vi "rpc_tsmaster_cmd_read_system_var.vi"(8 "error in (no error)":errorcluster caption="Incorrect input (no errors)", 9 "AHandle":i32, 10 "ASysVarName":string, 11 "Path input":path) -> (0 "error output":errorcluster, 1 "AHandle out":u32, 2 "return":i32, 3 "Path output":path, 4 "AValue":dbl)   [LabVIEW 2014]
doc: "Function introduction: Read system variables by name from remote TSMaster\nAfter calling the location to create TSMaster Rpc client\nInput parameter AHHandle: TSMaster Rpc client handle\nASysVarName: System variable name\nAValue: Data value pointer\nReturn value==0: Function execution successful\nOther values: Function execution failed"
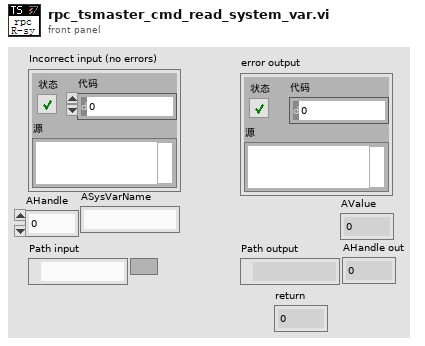
[diagram p1: front panel]
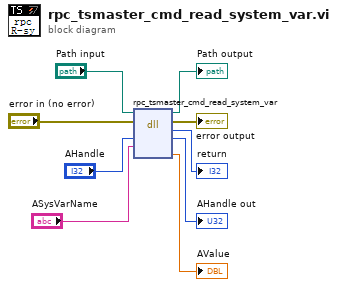
[diagram p0: block diagram]
diagram:
  n1 = dll-call lib="D:/Work/LabVIEW Code/TSMaster Labview SDK/LabVIEW/LabVIEW-TSMasterAPI_CLN/TSMasterAPI_LabVIEW-2024-10-08 14-20-13/Not_organized_vi/TSMaster.*" fn="rpc_tsmaster_cmd_read_system_var"(path in="Path input", error in="error in (no error)", "AHandle"="AHandle", "ASysVarName"="ASysVarName") -> (path out=→"Path output":path, error out=→"error output":errorcluster, "返回类型"=→"return":i32, "AHandle"=→"AHandle out":u32, "AValue"=→"AValue":dbl)  [unwired: 3 in]
